vi "Handle Command.vi"(8 "error in (no error)":errorcluster, 9 "Data":variant, 10 "Command":string, 11 "Inst.RP100 in":refnum<class "Inst.RP100.lvclass">) -> (0 "error out":errorcluster, 1 "Processed Data":variant, 2 "Command":string, 3 "Inst.RP100 out":refnum<class "Inst.RP100.lvclass">)   [LabVIEW 2019, in "Inst.RP100.lvclass"]
uses:
  Inst.RP100.lvclass
  Inst.RP100.lvclass/Inst.RP100.ctl
  Typedefs/getLevel--Cluster.ctl
  Typedefs/Channel--Num.ctl
  3a328603-7b30-4c06-b603-3c10f7f9975f.vi
  3a328603-7b30-4c06-b603-3c10f7f9975f.vi/1af63996-c7ff-464a-b6b6-1211024b9b29.vi
  3a328603-7b30-4c06-b603-3c10f7f9975f.vi/9682c448-3eb4-4c42-bbff-35e2f511437d.vi
  <vilib>/Utility/Data Type/Get Type Information.vi
  <vilib>/JDP Science/JSONtext/JSON text to Variant.vi
  <vilib>/JDP Science/JSONtext/LVClass Serializer/JSONtext LVClass Serializer.lvclass
  <userlib>/LevyLab/Instrument Framework/Instrument Types/Strain/Instrument.Strain.lvclass
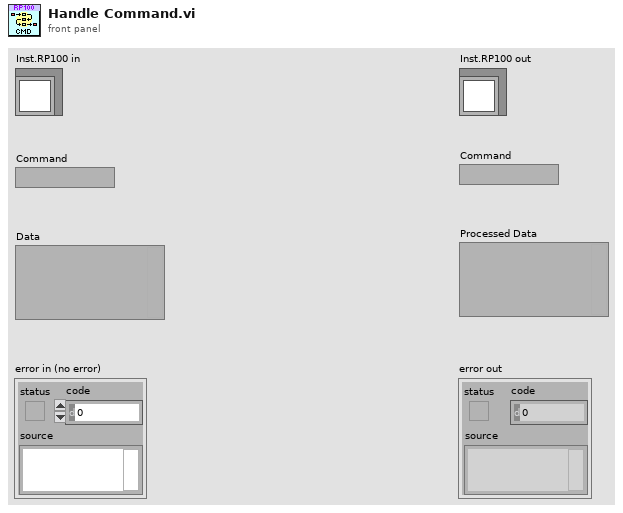
[diagram p1: front panel]
types:
  T1 = typedef "Inst.RP100.lvclass/getLevel--Cluster.ctl" = cluster{"Channel":T2}
  T2 = typedef "Inst.RP100.lvclass/Channel--Num.ctl" = i32
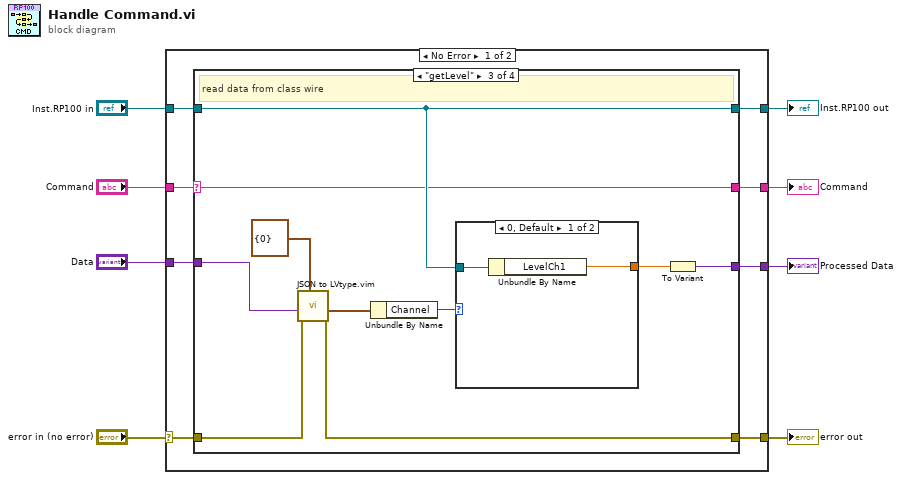
[diagram p0: block diagram]
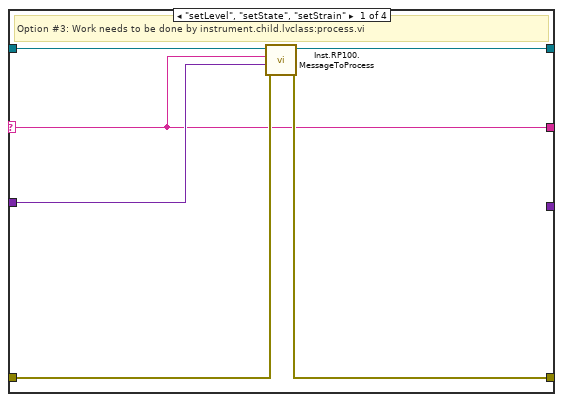
[diagram p2: hidden frame]
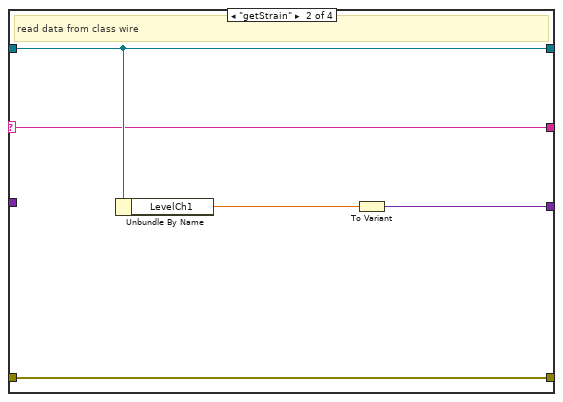
[diagram p3: hidden frame]
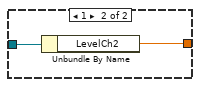
[diagram p4: hidden frame]
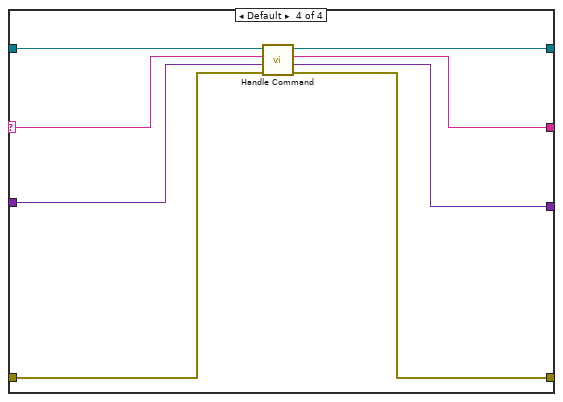
[diagram p5: hidden frame]
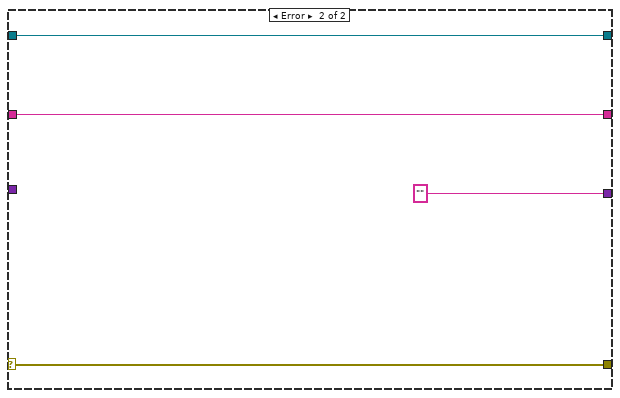
[diagram p6: hidden frame]
diagram:
  n1 = case shown="No Error" "error in (no error)" {
    selector: "error in (no error)" -> [w10 w53]
    tunnel: [w12 w53] -> w6
    tunnel: [w14 w52] -> w5
    tunnel: "Inst.RP100 in" -> [w15 w52]
    tunnel: "Command" -> [w16 w50]
    tunnel: [w13 "" ("String")] -> w3
    tunnel: "Data" -> [w9 _]
    tunnel: [w11 w50] -> w1
    frame No Error {
      n2 = case shown="\"getLevel\"" w16 {
        selector: w16 -> [w17 w23 w28 w43]
        tunnel: w15 -> [w22 w26 w35 w47]
        tunnel: [w21 w26 w35 w44] -> w14
        tunnel: [_ w25 w34 w46] -> w13
        tunnel: w10 -> [w20 w24 w31 w48]
        tunnel: w9 -> [w18 _ w32 w49]
        tunnel: [w19 w24 w30 w45] -> w12
        tunnel: [w17 w23 w28 w42] -> w11
        frame "setLevel", "setState", "setStrain" {
          # "Option #3: Work needs to be done by instrument.child.lvclass:process.vi"
          n3 = call "Inst.RP100.MessageToProcess.vi"("error in (no error)"=w20, "Data"=w18, "Command"=w17, "Inst.RP100 in"=w22) -> ("error out"=w19:errorcluster, "Inst.RP100 out"=w21:refnum<class "Inst.RP100.lvclass">)  [unwired: 6 in]
        }
        frame "getStrain" {
          # "read data from class wire"
          n4 = Unbundle By Name(w26) -> ("LevelCh1"=w27:dbl)
          n5 = To Variant(anything=w27) -> (Variant=w25:variant)
        }
        frame "getLevel" {
          # "read data from class wire"
          n6 = call "JSON to LVtype.vim"("type"=T1 {"Channel"=0} ("getLevel"), "error in (no error)"=w31, "JSON Data in"=w32) -> ("error out"=w30:errorcluster, "Data out"=w29:T1)  [unwired: 7 in]
          n7 = Unbundle By Name(w29) -> ("Channel"=w36:T2)
          n8 = case shown="0, Default" w36 {
            tunnel: [w39 w41] -> w37
            tunnel: w35 -> [w38 w40]
            frame 0, Default {
              n9 = Unbundle By Name(w38) -> ("LevelCh1"=w39:dbl)
            }
            frame 1 {
              n10 = Unbundle By Name(w40) -> ("LevelCh2"=w41:dbl)
            }
          }
          n11 = To Variant(anything=w37) -> (Variant=w34:variant)
        }
        frame Default {
          n12 = call-parent "Handle Command.vi"("error in (no error)"=w48, "params in"=w49, "command"=w43, "Instrument in"=w47) -> ("error out"=w45:errorcluster, "processed data"=w46:variant, "command out"=w42:string, "Instrument out"=w44:refnum<class "Inst.RP100.lvclass">)  [unwired: 4 in]
        }
      }
    }
    frame Error {
    }
  }
  "error out" <- w6
  "Inst.RP100 out" <- w5
  "Command" <- w1
  "Processed Data" <- w3
